vi "Create Message.vi"(7 "AppInst":refnum<vi>, 8 "error in (no error)":errorcluster, 9 "Destination Path":path, 10 "Actor class path":path, 11 "Message Maker in":refnum<class "Message Scripter.lvclass">) -> (0 "error out":errorcluster, 3 "Message Maker out":refnum<class "Message Scripter.lvclass">)   [LabVIEW 2020, in "Message Maker.lvlib" / "Message Scripter.lvclass"]
uses:
  Message Scripter.lvclass
  Message Scripter.lvclass/Message Scripter.ctl
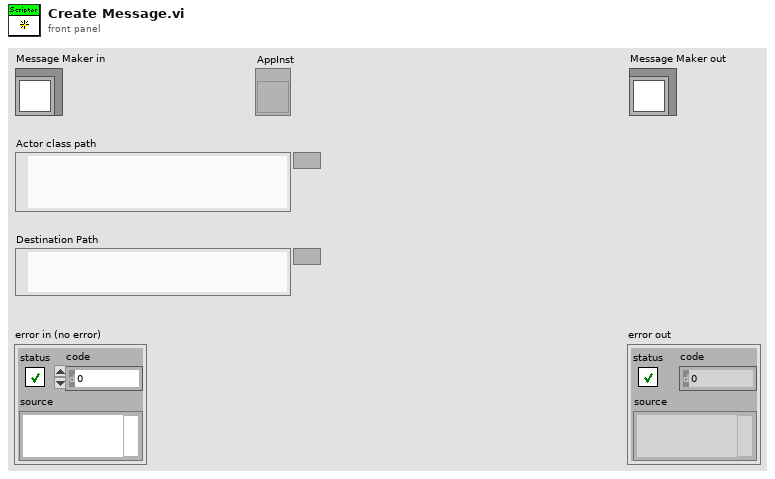
[diagram p1: front panel]
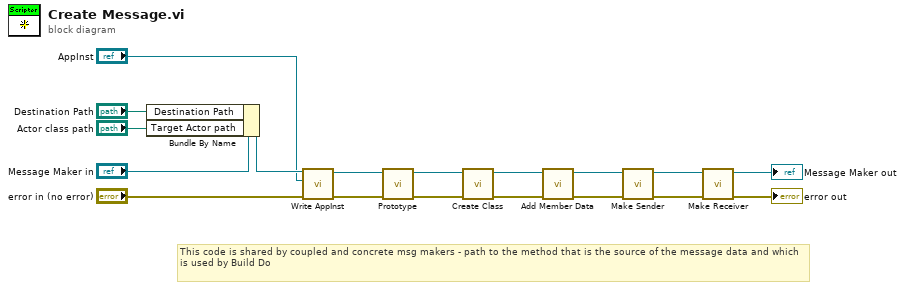
[diagram p0: block diagram]
diagram:
  # "This code is shared by coupled and concrete msg makers - path to the method that is the source of the message data and which is used by Build Do"
  n1 = Bundle By Name(cluster="Message Maker in", "Destination Path"="Destination Path", "Target Actor path"="Actor class path") -> (w15:refnum<class "Message Scripter.lvclass">)
  n2 = call "Write AppInst.vi"("error in (no error)"="error in (no error)", "AppInst"="AppInst", "Message Maker in"=w15) -> ("error out"=w14:errorcluster, "Message Maker out"=w11:refnum<class "Message Scripter.lvclass">)  [unwired: 7 in]
  n3 = call-dynamic "Prototype.vi"("error in (no error)"=w14, "Message Scripter in"=w11) -> ("error out"=w13:errorcluster, "Message Scripter out"=w12:refnum<class "Message Scripter.lvclass">)  [unwired: 8 in]
  n4 = call-dynamic "Create Class.vi"("error in (no error)"=w13, "Message Maker in"=w12) -> ("error out"=w9:errorcluster, "Message Maker out"=w10:refnum<class "Message Scripter.lvclass">)  [unwired: 8 in]
  n5 = call-dynamic "Add Member Data.vi"("error in (no error)"=w9, "Message Scripter in"=w10) -> ("error out"=w4:errorcluster, "Message Scripter out"=w3:refnum<class "Message Scripter.lvclass">)  [unwired: 8 in]
  n6 = call-dynamic "Make Sender.vi"("error in (no error)"=w4, "Message Scripter in"=w3) -> ("error out"=w2:errorcluster, "Message Scripter out"=w1:refnum<class "Message Scripter.lvclass">)  [unwired: 8 in]
  n7 = call-dynamic "Make Receiver.vi"("error in (no error)"=w2, "Message Scripter in"=w1) -> ("error out"=→"error out":errorcluster, "Message Scripter out"=→"Message Maker out":refnum<class "Message Scripter.lvclass">)  [unwired: 8 in]
